vi "Keithley-IV.vi"(0 "name":string="test", 1 "LED intensity":dbl=1.0) -> ()   [LabVIEW 2017]
uses:
  <vilib>/Utility/file.llb/Write Delimited Spreadsheet (DBL).vi
  Chunxiong Bao/Capacitance/Keithley 24XX/Keithley 24XX.lvlib
panel:
  in  "Record Voc":bool=TRUE
  in  "average":u32=3
  in  "LED":bool
  in  "string":string
  in  "Path":path=path "C:/Users/Biorgel/Documents/Data/Huotian/20190516_PM6_Y6_inverted_TemDep_Voclight"
  in  "IT Bias (V)":dbl
  out "T0":sgl
  in  "Measurement Speed (1 PLC)":dbl=1.0 format="%.2g"
  in  "stop":bool
  in  "IV/IT":bool
  in  "S":dbl=0.047
  in  "Compliance  Level (0.1)":dbl=0.1
  in  "VISA resource name":refnum<visa-resource-name>="GPIB0::25::INSTR"
  out "/J/-V":cluster{sgl[], dbl[]}(graph)
  out "J-V":cluster{dbl[], dbl[]}[](graph)
  in  "delay (ms)":dbl=50.0
  in  "cycle":dbl=0.5
  in  "step V":dbl=0.02
  in  "V":dbl=1.5
  in  "V0":dbl=-0.2
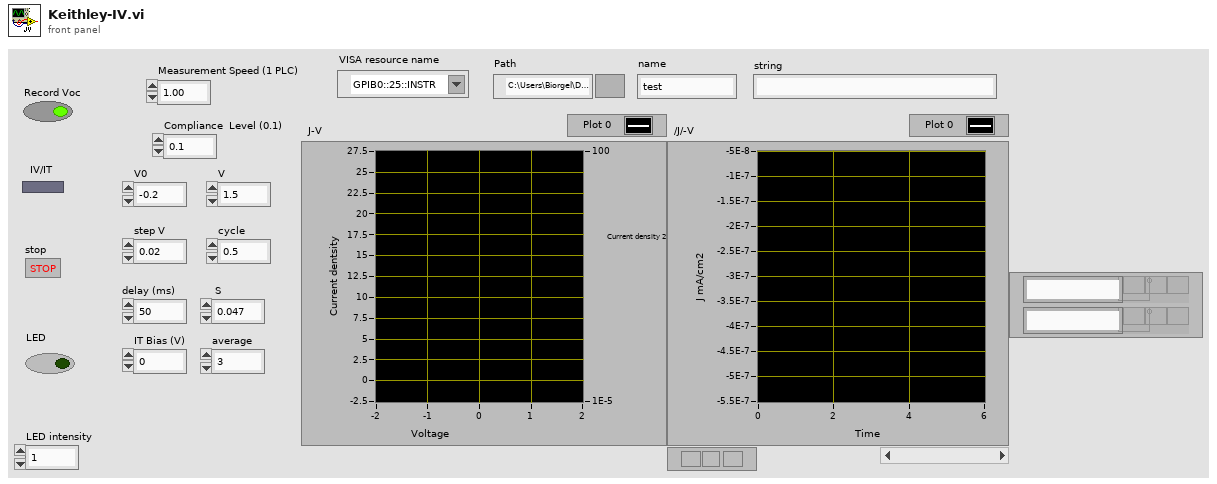
[diagram p1: front panel]
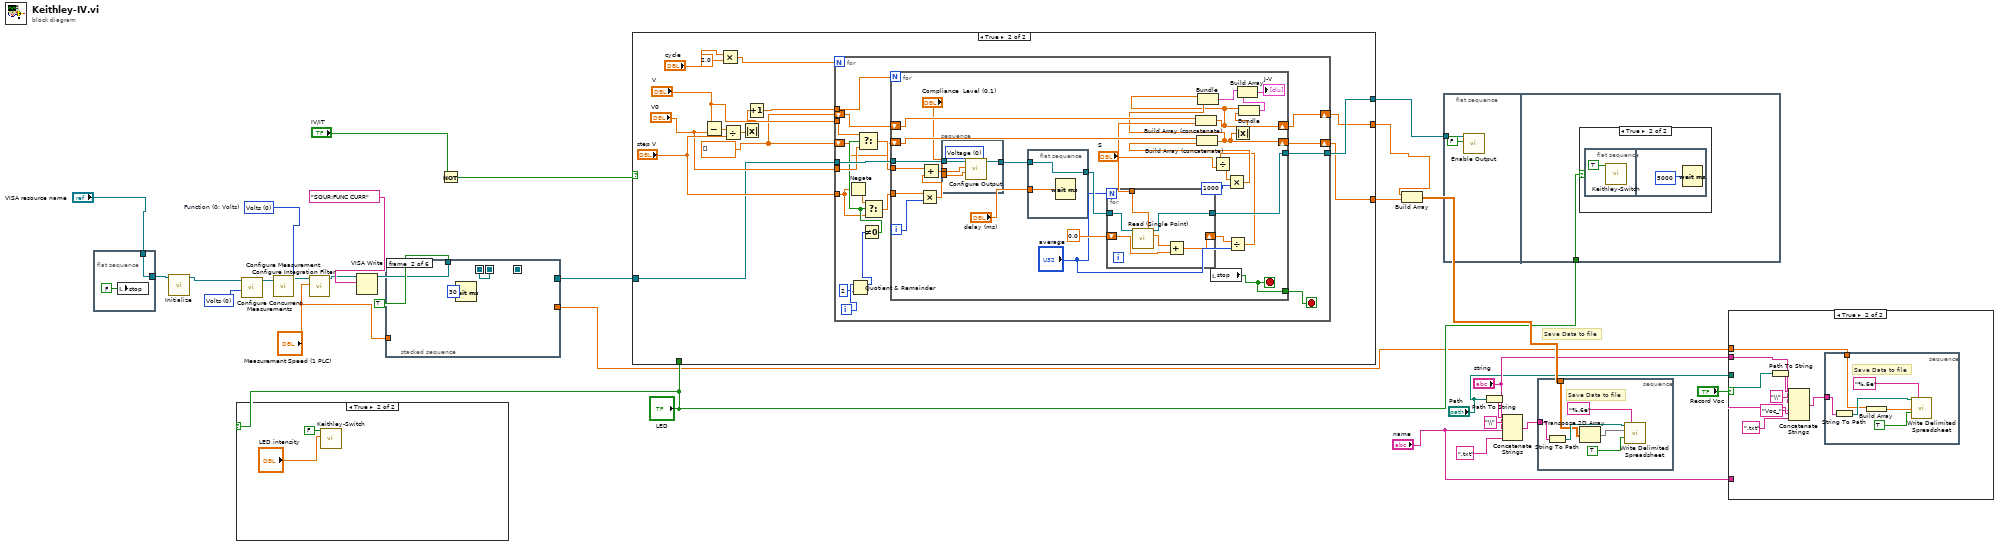
[diagram p0: block diagram]
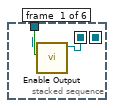
[diagram p3: hidden frame]
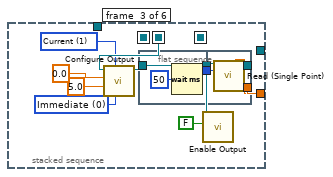
[diagram p4: hidden frame]
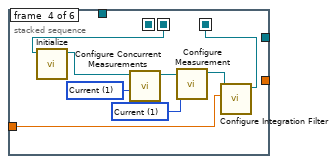
[diagram p5: hidden frame]
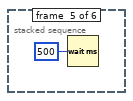
[diagram p6: hidden frame]
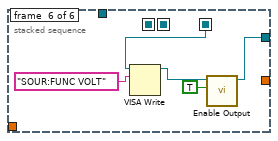
[diagram p7: hidden frame]
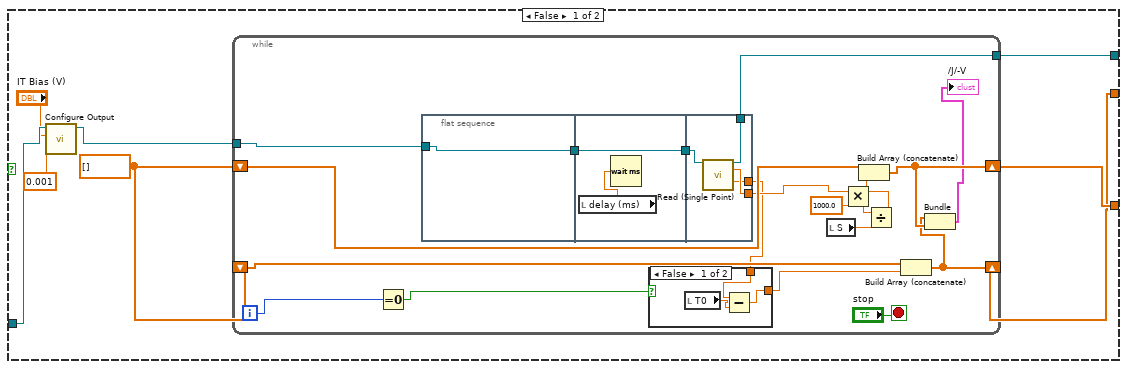
[diagram p10: hidden frame]
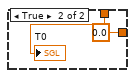
[diagram p11: hidden frame]
diagram:
  w24 = u16 0 items=["Volts", "Current", "Resistance", "Volt, Current", "Volts, Resistance", "Current, Resistance", "All"] ("Measurement Selection (3: Volts, Current)")
  w29 = u16 0 items=["Volts", "Current", "Resistance"]  # Function (0: Volts)
  # "Save Data to file"
  n1 = flat-sequence {
    tunnel: "VISA resource name" -> [w31]
    tunnel: [w31] -> w15
    frame #0 {
      n2 = local write "stop"(FALSE ("stop")) -> ()
    }
  }
  n3 = call <instrlib>:"Initialize.vi"("VISA resource name"=w15) -> ("VISA resource name out"=w23:refnum<visa-resource-name>)  [unwired: 9 in, 1 out]
  n4 = case shown="True" "LED" {
    frame False {
    }
    frame True {
      n5 = call "Keithley-Switch.vi"("SWITCH OFF"=FALSE, "Gain"="LED intensity") -> ()  [unwired: 9 in]
    }
  }
  n6 = call "Configure Concurrent Measurements.vi"("Measurement Selection (3: Volts, Current)"=w24, "VISA resource name"=w23) -> ("VISA resource name out"=w25:refnum<visa-resource-name>)  [unwired: 8 in, 1 out]
  n7 = call "Configure Measurement.vi"("Function (0: Volts)"=w29, "VISA resource name"=w25) -> ("VISA resource name out"=w20:refnum<visa-resource-name>)  [unwired: 8 in, 1 out]
  n8 = call <instrlib>:"Configure Integration Filter.vi"("Measurement Speed (1 PLC)"="Measurement Speed (1 PLC)", "VISA resource name"=w20) -> ("VISA resource name out"=w19:refnum<visa-resource-name>)  [unwired: 8 in, 1 out]
  n9 = VISA Write(VISA resource name=w19, write buffer="SOUR:FUNC CURR" ("multi-line string")) -> (VISA resource name out=w22:refnum<visa-resource-name>)  [unwired: 1 in, 2 out]
  n10 = stacked-sequence {
    seq-local: [w36 _ _ _ _ _] -> [_ w38 _ _ _ _]
    seq-local: [_ w38 _ _ _ _] -> [_ _ w49 w61 _ _]
    seq-local: [_ _ _ w57 _ _] -> [_ _ _ _ _ w69]
    tunnel: TRUE ("Enable Output (T: Enable)") -> [w35 _ _ _ _ _]
    tunnel: w22 -> [w34 _ _ _ _ _]
    tunnel: [_ _ _ _ _ w67] -> w28
    tunnel: [_ _ w44 _ _ _] -> w2
    tunnel: "Measurement Speed (1 PLC)" -> [_ _ _ w58 _ _]
    frame #0 {
      n11 = call "Enable Output.vi"("Enable Output (T: Enable)"=w35, "VISA resource name"=w34) -> ("VISA resource name out"=w36:refnum<visa-resource-name>)  [unwired: 8 in, 1 out]
    }
    frame #1 {
      n12 = Wait (ms)(milliseconds to wait=u32 30) -> ()  [unwired: 1 out]
    }
    frame #2 {
      w46 = u16 0 items=["Immediate", "Triggered"] ("Output Type  (0: Immediate)")
      w48 = u16 1 items=["Voltage", "Current"] ("Source Mode  (0: Voltage)")
      n13 = call "Configure Output.vi"("Output Type  (0: Immediate)"=w46, "Source Mode  (0: Voltage)"=w48, "Compliance  Level (0.1)"=5.0, "Output Level (0)"=0.0, "VISA resource name"=w49) -> ("VISA resource name out"=w45:refnum<visa-resource-name>)  [unwired: 5 in, 1 out]
      n14 = flat-sequence {
        tunnel: w45 -> [w52]
        tunnel: [w52] -> w41
        tunnel: [w51] -> w40
        tunnel: [w55] -> w44
        tunnel: [w54] -> w43
        tunnel: w41 -> [w56]
        tunnel: w40 -> [w53]
        frame #0 {
          n15 = Wait (ms)(milliseconds to wait=u32 50) -> (millisecond timer value=w51:u32)
        }
        frame #1 {
          n16 = call "Read (Single Point).vi"("VISA resource name"=w56, "Timeout (10000 ms)"=w53) -> ("Voltage"=w55:sgl, "VISA resource name out"=w54:refnum<visa-resource-name>)  [unwired: 7 in, 5 out]
        }
      }
      n17 = call "Enable Output.vi"("Enable Output (T: Enable)"=FALSE, "VISA resource name"=w43) -> ()  [unwired: 8 in, 2 out]
    }
    frame #3 {
      w62 = u16 1 items=["Volts", "Current", "Resistance"] ("Function (0: Volts)")
      w63 = u16 1 items=["Volts", "Current", "Resistance", "Volt, Current", "Volts, Resistance", "Current, Resistance", "All"] ("Measurement Selection (3: Volts, Current)")
      n18 = call <instrlib>:"Initialize.vi"("VISA resource name"=w61) -> ("VISA resource name out"=w60:refnum<visa-resource-name>)  [unwired: 9 in, 1 out]
      n19 = call "Configure Concurrent Measurements.vi"("Measurement Selection (3: Volts, Current)"=w63, "VISA resource name"=w60) -> ("VISA resource name out"=w64:refnum<visa-resource-name>)  [unwired: 8 in, 1 out]
      n20 = call "Configure Measurement.vi"("Function (0: Volts)"=w62, "VISA resource name"=w64) -> ("VISA resource name out"=w59:refnum<visa-resource-name>)  [unwired: 8 in, 1 out]
      n21 = call <instrlib>:"Configure Integration Filter.vi"("Measurement Speed (1 PLC)"=w58, "VISA resource name"=w59) -> ("VISA resource name out"=w57:refnum<visa-resource-name>)  [unwired: 8 in, 1 out]
    }
    frame #4 {
      n22 = Wait (ms)(milliseconds to wait=u32 500) -> ()  [unwired: 1 out]
    }
    frame #5 {
      n23 = VISA Write(VISA resource name=w69, write buffer="SOUR:FUNC VOLT" ("multi-line string")) -> (VISA resource name out=w68:refnum<visa-resource-name>)  [unwired: 1 in, 2 out]
      n24 = call "Enable Output.vi"("Enable Output (T: Enable)"=TRUE, "VISA resource name"=w68) -> ("VISA resource name out"=w67:refnum<visa-resource-name>)  [unwired: 8 in, 1 out]
    }
  }
  n25 = Not(x="IV/IT") -> (.not. x?=w17:bool)
  n26 = case shown="True" w17 {
    tunnel: w28 -> [w74 w120]
    tunnel: [w77 w112] -> w26
    tunnel: [w75 w111] -> w7
    tunnel: [w76 w110] -> w6
    tunnel: "LED" -> [_ _]
    frame False {
      w78 = sgl[] []
      n27 = call "Configure Output.vi"("Compliance  Level (0.1)"=0.001, "Output Level (0)"="IT Bias (V)", "VISA resource name"=w74) -> ("VISA resource name out"=w73:refnum<visa-resource-name>)  [unwired: 7 in, 1 out]
      n28 = while {
        tunnel: w73 -> [w95]
        shift-right: [w91] -> w76
        shift-left: w78 -> [w92]
        shift-right: [w90] -> w75
        shift-left: w78 -> [w93]
        tunnel: [w89] -> w77
        i -> [w82]
        stop <- "stop" stop-if-true
        n29 = Equal To 0?(x=w82) -> (x = 0?=w81:bool)
        n30 = flat-sequence {
          tunnel: [w103] -> w97
          tunnel: w95 -> [w103]
          tunnel: [w104] -> w96
          tunnel: w97 -> [w104]
          tunnel: w96 -> [w109]
          tunnel: [w108] -> w84
          tunnel: [w107] -> w89
          tunnel: [w106] -> w80
          frame #0 {
          }
          frame #1 {
            n31 = local read "delay (ms)"() -> (w105:dbl)
            n32 = Wait (ms)(milliseconds to wait=w105) -> ()  [unwired: 1 out]
          }
          frame #2 {
            n33 = call "Read (Single Point).vi"("VISA resource name"=w109) -> ("VISA resource name out"=w107:refnum<visa-resource-name>, "Current"=w108:sgl, "Timestamp"=w106:sgl)  [unwired: 8 in, 4 out]
          }
        }
        n34 = case shown="False" w81 {
          tunnel: w80 -> [w99 w102]
          tunnel: [w100 sgl 0.0] -> w79
          frame False {
            n35 = local read "T0"() -> (w98:sgl)
            n36 = Subtract(x=w99, y=w98) -> (x-y=w100:sgl)
          }
          frame True {
            "T0" <- w102
          }
        }
        n37 = local read "S"() -> (w87:dbl)
        n38 = Multiply(x=w84, y=1000.0) -> (x*y=w86:dbl)
        n39 = Divide(x=w86, y=w87) -> (x/y=w88:dbl)
        n40 = Build Array (concatenate)(w92, w88) -> (w91:dbl[])
        n41 = Build Array (concatenate)(w93, w79) -> (w90:sgl[])
        n42 = Bundle(w90, w91) -> (→"/J/-V":cluster{sgl[], dbl[]})  [unwired: 1 in]
      }
    }
    frame True {
      w115 = dbl[] []
      n43 = Subtract(x="V", y="V0") -> (x-y=w124:dbl)
      n44 = Multiply(x="cycle", y=2.0) -> (x*y=w117:dbl)
      n45 = Divide(x=w124, y="step V") -> (x/y=w114:dbl)
      n46 = Absolute Value(x=w114) -> (abs(x)=w113:dbl)
      n47 = Increment(x=w113) -> (x+1=w121:dbl)
      n48 = for {
        N: w117 -> [_]
        tunnel: "step V" -> [w131]
        tunnel: "V0" -> [w137]
        tunnel: w121 -> [w142]
        tunnel: w120 -> [w141]
        tunnel: "V" -> [w138]
        shift-right: [w130] -> w111
        shift-left: w115 -> [w129]
        shift-right: [w128] -> w110
        shift-left: w115 -> [w127]
        tunnel: [w126] -> w112
        i -> [w140]
        stop <- w125 stop-if-true
        n49 = Negate(x=w131) -> (-x=w132:dbl)
        n50 = Quotient & Remainder(x=w140, y=2) -> (x-y*floor(x/y)=w134:i32)  [unwired: 1 out]
        n51 = Not Equal To 0?(x=w134) -> (x != 0?=w133:bool)
        n52 = Select(t=w138, s=w133, f=w137) -> (s? t:f=w136:dbl)
        n53 = Select(t=w132, s=w133, f=w131) -> (s? t:f=w135:dbl)
        n54 = for {
          N: w142 -> [_]
          tunnel: w135 -> [w170]
          tunnel: w136 -> [w168]
          tunnel: w141 -> [w151]
          shift-right: [w158] -> w128
          shift-left: w127 -> [w162]
          shift-right: [w157] -> w130
          shift-left: w129 -> [w160]
          tunnel: [w152] -> w126
          tunnel: [w147] -> w125
          i -> [w171]
          stop <- w147 stop-if-true
          n55 = Multiply(x=w170, y=w171) -> (x*y=w169:dbl)
          n56 = Add(x=w168, y=w169) -> (x+y=w149:dbl)
          n57 = stacked-sequence {
            tunnel: w151 -> [w176]
            tunnel: [w175] -> w150
            tunnel: w149 -> [w174]
            tunnel: "Compliance  Level (0.1)" -> [w173]
            frame #0 {
              w172 = u16 0 items=["Voltage", "Current"] ("Source Mode  (0: Voltage)")
              n58 = call "Configure Output.vi"("Source Mode  (0: Voltage)"=w172, "Compliance  Level (0.1)"=w173, "Output Level (0)"=w174, "VISA resource name"=w176) -> ("VISA resource name out"=w175:refnum<visa-resource-name>)  [unwired: 6 in, 1 out]
            }
          }
          n59 = flat-sequence {
            tunnel: w150 -> [w184]
            tunnel: [w184] -> w167
            tunnel: "delay (ms)" -> [w183]
            frame #0 {
              n60 = Wait (ms)(milliseconds to wait=w183) -> ()  [unwired: 1 out]
            }
          }
          n61 = for {
            N: "average" -> [_]
            tunnel: [w181] -> w161
            tunnel: w167 -> [w182]
            tunnel: [w180] -> w152
            shift-right: [w177] -> w145
            shift-left: 0.0 -> [w179]
            n62 = call "Read (Single Point).vi"("VISA resource name"=w182) -> ("Voltage"=w181:sgl, "VISA resource name out"=w180:refnum<visa-resource-name>, "Current"=w178:sgl)  [unwired: 8 in, 4 out]
            n63 = Add(x=w178, y=w179) -> (x+y=w177:dbl)
          }
          n64 = Build Array (concatenate)(w160, w161) -> (w157:dbl[])
          n65 = local read "stop"() -> (w147:bool)
          n66 = Divide(x=w145, y="average") -> (x/y=w143:dbl)
          n67 = Divide(x=w143, y="S") -> (x/y=w164:dbl)
          n68 = Multiply(x=w164, y=1000) -> (x*y=w163:dbl)
          n69 = Build Array (concatenate)(w162, w163) -> (w158:dbl[])
          n70 = Bundle(w157, w158) -> (w155:cluster{dbl[], dbl[]})  [unwired: 1 in]
          n71 = Absolute Value(x=w158) -> (abs(x)=w156:dbl[])
          n72 = Bundle(w157, w156) -> (w154:cluster{dbl[], dbl[]})  [unwired: 1 in]
          n73 = Build Array(w155, w154) -> (→"J-V":cluster{dbl[], dbl[]}[])
        }
      }
    }
  }
  n74 = Build Array(w7, w6) -> (w12:dbl[][])
  n75 = flat-sequence {
    tunnel: w26 -> [w186]
    tunnel: "LED" -> [w187]
    frame #0 {
      n76 = call "Enable Output.vi"("Enable Output (T: Enable)"=FALSE, "VISA resource name"=w186) -> ()  [unwired: 8 in, 2 out]
    }
    frame #1 {
      n77 = case shown="True" w187 {
        frame False {
        }
        frame True {
          n78 = flat-sequence {
            frame #0 {
              n79 = call "Keithley-Switch.vi"("SWITCH OFF"=TRUE) -> ()  [unwired: 10 in]
            }
            frame #1 {
              n80 = Wait (ms)(milliseconds to wait=u32 5000) -> ()  [unwired: 1 out]
            }
          }
        }
      }
    }
  }
  n81 = Path To String(path="Path") -> (string=w11:string)
  n82 = Concatenate Strings(w11, "\\" ("string"), "string", "name", ".txt" ("string")) -> (w13:string)
  n83 = stacked-sequence {
    tunnel: w12 -> [w191]
    tunnel: w13 -> [w194]
    frame #0 {
      # "Save Data to file"
      n84 = String To Path(string=w194) -> (path=w193:path)
      n85 = Transpose 2D Array(2D array=w191) -> (transposed array=w190:dbl[][])
      n86 = call-poly <vilib>:"Write Delimited Spreadsheet.vi"("file path (dialog if empty)"=w193, "format (%.3f)"="%.6e", "2D data"=w190, "append to file? (new file:F)"=TRUE) -> ()  [unwired: 10 in, 2 out]
    }
  }
  n87 = case shown="True" "Record Voc" {
    tunnel: "string" -> [_ w201]
    tunnel: "Path" -> [_ w200]
    tunnel: "name" -> [_ w198]
    tunnel: w2 -> [_ w196]
    frame False {
    }
    frame True {
      n88 = Path To String(path=w200) -> (string=w202:string)
      n89 = Concatenate Strings(w202, "\\" ("string"), w201, "Voc_" ("string"), w198, ".txt" ("string")) -> (w203:string)
      n90 = stacked-sequence {
        tunnel: w196 -> [w206]
        tunnel: w203 -> [w209]
        frame #0 {
          # "Save Data to file"
          n91 = String To Path(string=w209) -> (path=w208:path)
          n92 = Build Array(w206) -> (w205:sgl[])
          n93 = call-poly <vilib>:"Write Delimited Spreadsheet.vi"("file path (dialog if empty)"=w208, "format (%.3f)"="%.6e", "1D data"=w205, "append to file? (new file:F)"=TRUE) -> ()  [unwired: 10 in, 2 out]
        }
      }
    }
  }
